vi "Drive Controller.vi"(8 "error in":errorcluster) -> ()   [LabVIEW 2017]
doc: "This VI executes continuously carrying out the current operation and responding to updates or new operation requests. It will often contain the timing or control code that is difficult to place directly in TeleOp. This VI generally opens all sensors and motors and isolates the rest of the robot code from knowing implementation details of how the operations are carried out."
uses:
  Drive Operations.ctl
  Drive Setpoints.ctl
  <vilib>/Rock Robotics/WPI/SafetyOutput/WPI_SafetyOutputConfigMenu.ctl
  <vilib>/Rock Robotics/WPI/RobotDrive/WPI_RobotDriveMecanumDrive_Cartesian.vi
  <vilib>/Rock Robotics/WPI/Framework/Completion Status.ctl
panel:
  in  "Interactive Values":T1
  in  "Buttons":cluster{"Execute Cmd":bool, "Abort Cmd":bool}
  out "Command Timing":cluster{"Start Time (ms)":u32, "Iterations":i32}
  out "Status":T3
  out "Setpoints":T4(graph)
  out "Current\nCmd":string
  # "Tip: The graph shows the motor setpoints. It may also be helpful to observe inputs and sensor values.\nYou may also want to display tuning or debugging controls."
  # "Interactive Command: You may fill in the settings for a command\nand schedule it with the Execute button. You can observe and abort\nany command while fine tuning the code for the controller."
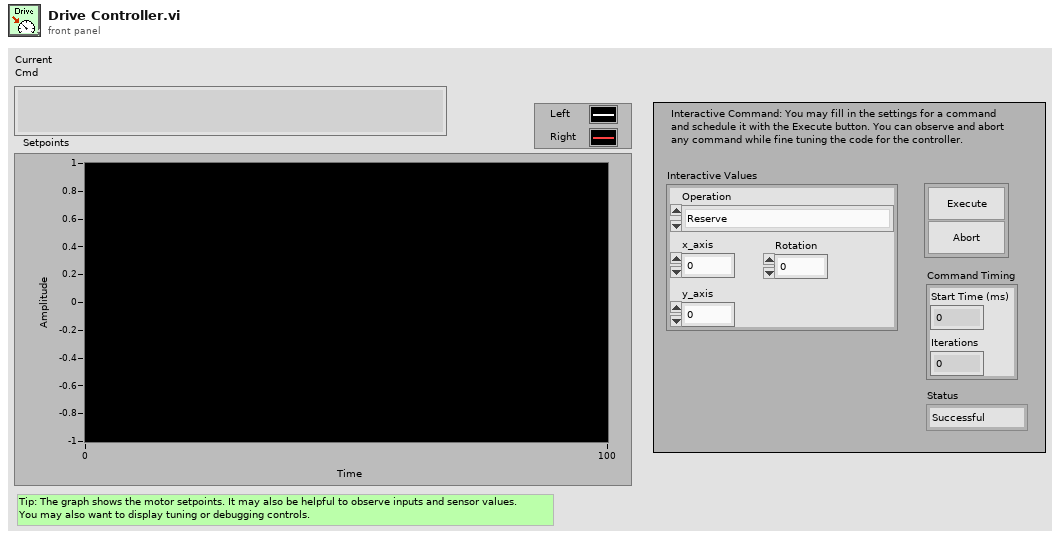
[diagram p1: front panel]
types:
  T1 = typedef "Drive Setpoints.ctl" = cluster{"Operation":T2, "x_axis":dbl, "Rotation":dbl, "y_axis":dbl}
  T2 = typedef "Drive Operations.ctl" = enum16{"Reserve", "Read Current", "Immediate", "Drive for Time", "Drive for Distance"}
  T3 = typedef "Completion Status.ctl" = enum16{"Successful", "Aborted", "Incomplete"}
  T4 = cluster{"Left Setpoint":dbl, "Right Setpoint":dbl}
  T5 = typedef "WPI_SafetyOutputConfigMenu.ctl" = enum16{"Enable", "Disable"}
  T6 = typedef "Command Status Info.ctl" = cluster{"Name":string, "Status":T3, "notifier out":T7}
  T7 = typedef "Completion Notifier.ctl" = refnum<notifier>
  T8 = cluster{"SubSystem Data":T1, cluster{"Start Time (ms)":u32, "Iterations":i32}, cluster{"Command Info":T6, "Description":string, "Default Command":T1, "queue out":refnum<queue>, "Subsystem Name":string}}
  T9 = typedef "WPI_RobotDriveDevRef.ctl" = cluster{"DevStatus":errorcluster, "Motors[]":T10[], "Square Inputs":bool, "Max Output":dbl}
  T10 = typedef "WPI_MotorControlDeviceRef.ctl" = cluster{"DeviceStatus":errorcluster, "Type":T11, "PWM":cluster{"PWM Channel":T12, "DeadBand":T13}, "CAN":cluster{"Device Number":u8, "SetOutput VI Ref":variant, "GetOutput VI Ref":variant, "Enable VI Ref":variant, "Disable VI Ref":variant, "Data":variant}, "Invert":bool, "DIO PWM":cluster{"PWM \"Enable\" Channel":T12, "DIOChannel":T14, "PWM Rate":dbl}}
  T11 = typedef "WPI_MotorControlType.ctl" = enum16{"PWM", "CAN", "DIO PWM"}
  T12 = typedef "FPGA_DIOPWMChannel.ctl" = enum8{"PWM 0", "PWM 1", "PWM 2", "PWM 3", "PWM 4", "PWM 5", "PWM 6", "PWM 7", "PWM 8", "PWM 9", "PWM MXP 0", "PWM MXP 1", "PWM MXP 2", "PWM MXP 3", "PWM MXP 4", "PWM MXP 5", "PWM MXP 6", "PWM MXP 7", "PWM MXP 8", "PWM MXP 9", "Invalid"}
  T13 = typedef "WPI_PWMDeadband.ctl" = cluster{"Name":string, "maxPositivePwm":i32, "minPositivePwm":i32, "centerPwm":i32, "maxNegativePwm":i32, "minNegativePwm":i32, "angularRange":u16}
  T14 = typedef "FPGA_DIOChannel.ctl" = enum8{"DIO 0", "DIO 1", "DIO 2", "DIO 3", "DIO 4", "DIO 5", "DIO 6", "DIO 7", "DIO 8", "DIO 9", "DIO MXP 0", "DIO MXP 1", "DIO MXP 2", "DIO MXP 3", "DIO MXP 4", "DIO MXP 5", "DIO MXP 6", "DIO MXP 7", "DIO MXP 8", "DIO MXP 9", "DIO MXP 10", "DIO MXP 11", "DIO MXP 12", "DIO MXP 13", "DIO MXP 14", "DIO MXP 15", "SPI Port CS1", "SPI Port CS2", "SPI Port CS3", "SPI Port MISO", "SPI Port MOSI", "Invalid"}
  T15 = cluster{"SubSystem Data":T1, cluster{"Start Time (ms)":u32, "Iterations":i32}, "Default Command Arguments":cluster{"Command Info":T6, "Description":string, "Default Command":T1, "queue out":refnum<queue>, "Subsystem Name":string}}
  T16 = cluster{"Don't move motors while reserved":dbl, "Don't move motors while reserved":dbl}
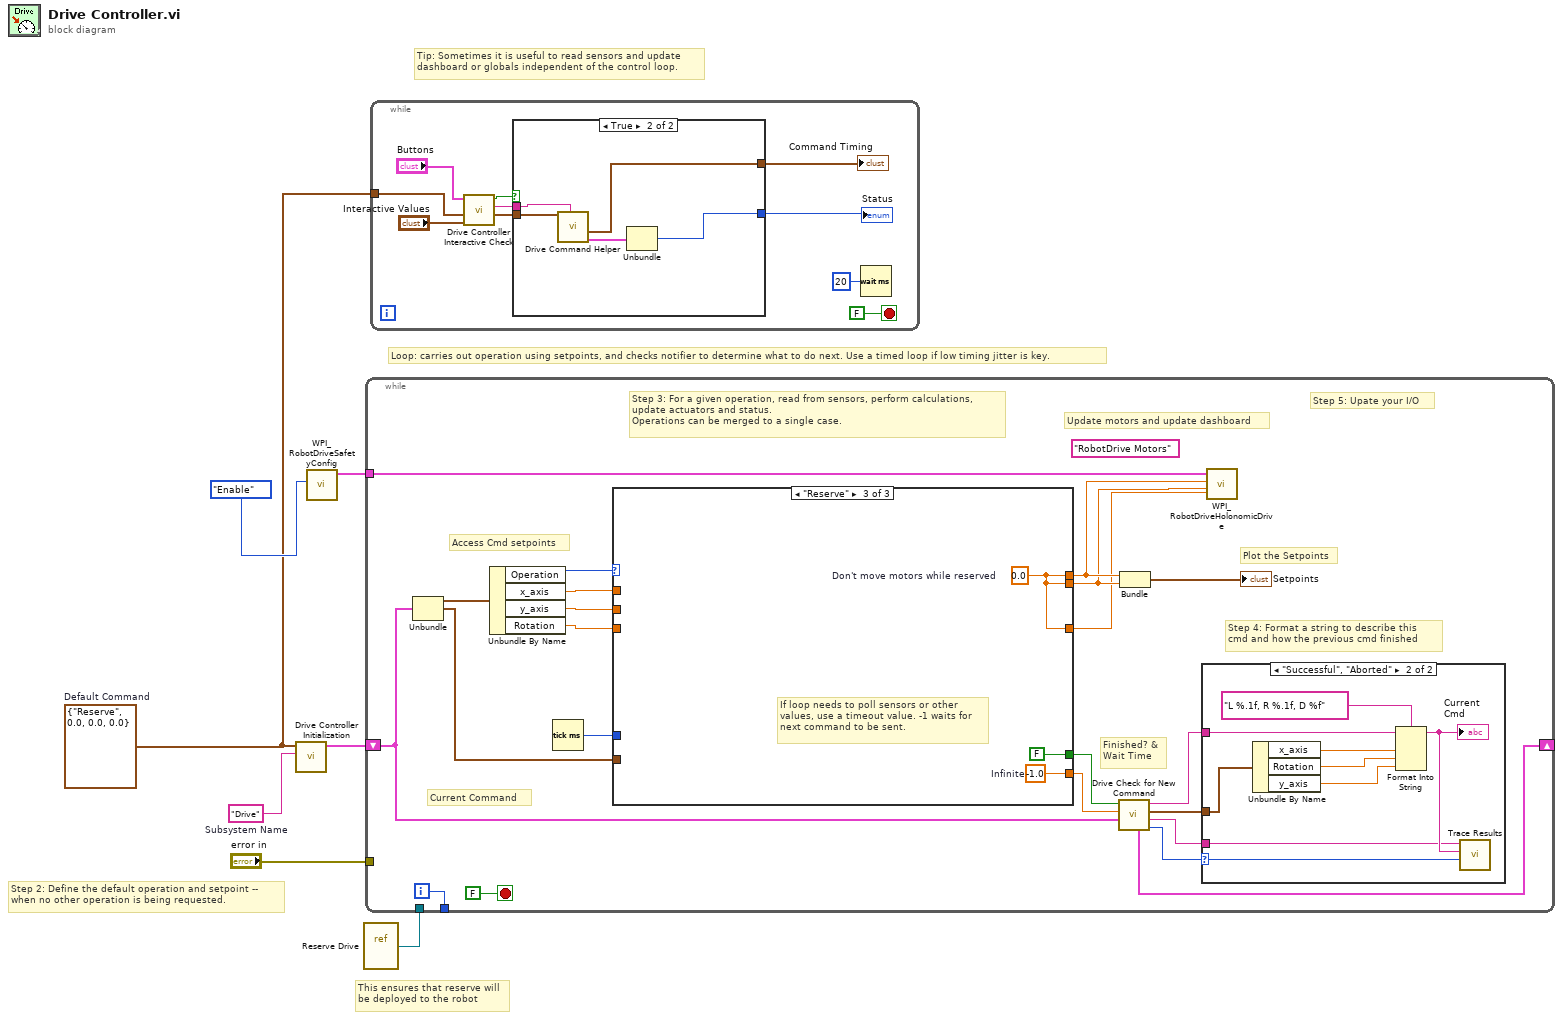
[diagram p0: block diagram]
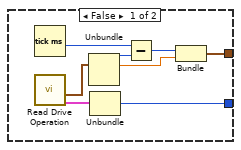
[diagram p2: hidden frame]
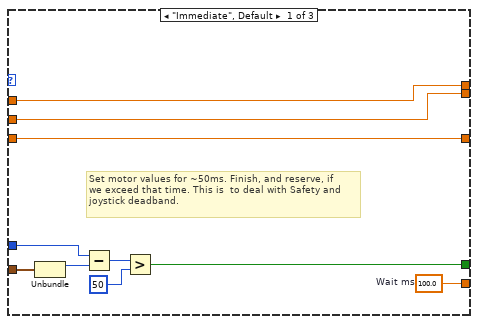
[diagram p4: hidden frame]
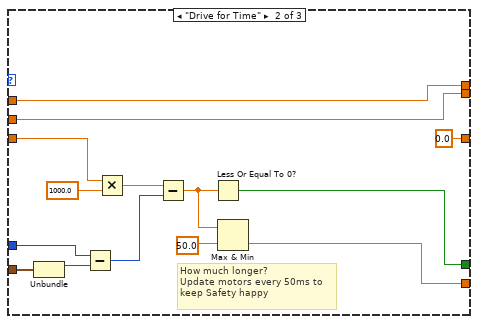
[diagram p5: hidden frame]
diagram:
  w2 = T1 {"Operation"=enum."Reserve", "x_axis"=0.0, "Rotation"=0.0, "y_axis"=0.0}  # Default Command
  w8 = "Drive"  # Subsystem Name
  # "This ensures that reserve will\nbe deployed to the robot"
  # "Tip: Sometimes it is useful to read sensors and update\ndashboard or globals independent of the control loop."
  # "Step 2: Define the default operation and setpoint --\nwhen no other operation is being requested."
  # "Loop: carries out operation using setpoints, and checks notifier to determine what to do next. Use a timed loop if low timing jitter is key."
  n1 = call "Drive Controller Initialization.vi"("Subsystem Name"=w8, "Default Command"=w2) -> ("Current Command"=w4:T8)  [unwired: 9 in]
  n2 = call <vilib>:"WPI_RobotDriveSafetyConfig.vi"("mode"=WPI_SafetyOutputConfigMenu."Enable") -> (3:"RobotDriveDevRef"=w6:T9, 11:"RobotDriveDevRef"=w1:T9)  [unwired: 8 in, 1 out]
  n3 = vi-ref "Reserve Drive.vi"() -> (w3:refnum<vi>)
  n4 = while {
    shift-right: [w20] -> _
    shift-left: w4 -> [w13]
    tunnel: [w29] -> _
    tunnel: w6 -> [w12]
    tunnel: "error in" -> [_]
    tunnel: w3 -> [_]
    i -> [w29]
    stop <- FALSE stop-if-true
    (unwired) "RobotDrive Motors" ("Name")
    # "Step 5: Upate your I/O"
    # "Step 4: Format a string to describe this\ncmd and how the previous cmd finished"
    # "Current Command"
    # "Update motors and update dashboard"
    # "Plot the Setpoints"
    # "Access Cmd setpoints"
    # "Finished? &\nWait Time"
    # "Step 3: For a given operation, read from sensors, perform calculations,\nupdate actuators and status.\nOperations can be merged to a single case."
    n5 = Unbundle(w13) -> ("SubSystem Data"=w27:T1, w14:cluster{"Start Time (ms)":u32, "Iterations":i32})  [unwired: 1 out]
    n6 = Unbundle By Name(w27) -> ("Operation"=w26:T2, "x_axis"=w25:dbl, "y_axis"=w24:dbl, "Rotation"=w23:dbl)
    n7 = Tick Count (ms)() -> (millisecond timer value=w22:u32)
    n8 = case shown="\"Reserve\"" w26 {
      tunnel: [w49 w51 w66] -> w19
      tunnel: [w42 w58 FALSE ("ignore previous (F)")] -> w18
      tunnel: w14 -> [w41 w60 _]
      tunnel: [w48 w57 w64] -> w11
      tunnel: [w47 w56 w64] -> w10
      tunnel: w25 -> [w48 w57 _]
      tunnel: w24 -> [w47 w56 _]
      tunnel: w23 -> [w40 w55 _]
      tunnel: w22 -> [w43 w54 _]
      tunnel: [w40 0.0 ("Rotation") w64] -> w9
      frame "Immediate", Default {
        w49 = 100.0  # Wait ms
        # "Set motor values for ~50ms. Finish, and reserve, if\nwe exceed that time. This is  to deal with Safety and\njoystick deadband."
        n9 = Unbundle(w41) -> ("Start Time (ms)"=w44:u32)  [unwired: 1 out]
        n10 = Subtract(x=w43, y=w44) -> (x-y=w45:u32)
        n11 = Greater?(x=w45, y=u8 50 ("Left Motor")) -> (0:w42:bool)
      }
      frame "Drive for Time" {
        # "How much longer?\nUpdate motors every 50ms to\nkeep Safety happy"
        n12 = Unbundle(w60) -> ("Start Time (ms)"=w59:u32)  [unwired: 1 out]
        n13 = Subtract(x=w54, y=w59) -> (x-y=w63:u32)
        n14 = Multiply(x=w55, y=1000.0) -> (x*y=w62:dbl)
        n15 = Subtract(x=w62, y=w63) -> (x-y=w53:dbl)
        n16 = Less Or Equal To 0?(x=w53) -> (x <= 0?=w58:bool)
        n17 = Max & Min(x=w53, y=50.0) -> (min(x,y)=w51:dbl)  [unwired: 1 out]
      }
      frame "Reserve" {
        w64 = 0.0  # Don't move motors while reserved
        w66 = -1.0  # Infinite
        # "If loop needs to poll sensors or other\nvalues, use a timeout value. -1 waits for\nnext command to be sent."
      }
    }
    n18 = call "Drive Check for New Command.vi"("input cluster"=w13, "Wait time (ms)"=w19, "Finished?"=w18) -> ("Completion"=w21:T3, "Subsystem Name"=w15:string, "Current Command"=w16:T1, "Initial Trace String"=w17:string, "Next Command"=w20:T15)  [unwired: 4 in]
    n19 = Bundle("Don't move motors while reserved"=w11, "Don't move motors while reserved"=w10) -> (→"Setpoints":T16)  [unwired: 1 in]
    n20 = case shown="\"Successful\", \"Aborted\"" w21 {
      selector: w21 -> [_ w39]
      tunnel: w17 -> [_ w34]
      tunnel: w16 -> [_ w35]
      tunnel: w15 -> [_ w31]
      frame "Incomplete", Default {
        # "Continuing current command"
      }
      frame "Successful", "Aborted" {
        # "Report and setup for next command"
        n21 = Unbundle By Name(w35) -> ("x_axis"=w37:dbl, "Rotation"=w38:dbl, "y_axis"=w32:dbl)
        n22 = Format Into String(format string="L %.1f, R %.1f, D %f", initial string=w34, w37, w38, w32) -> (resulting string=w33:string)  [unwired: 1 in, 1 out]
        "Current\nCmd" <- w33
        n23 = call <vilib>:"Trace Results.vi"("Status of previous command"=w39, "Description"=w33, "Subsystem"=w31) -> ()  [unwired: 9 in]
      }
    }
    n24 = call-poly <vilib>:"WPI_RobotDriveHolonomicDrive.vi"("Rotation"=w9, "Y"=w10, "X"=w11, "RobotDriveDevRef"=w12) -> ()  [unwired: 5 in, 3 out]
  }
  n25 = while {
    tunnel: w2 -> [w68]
    stop <- FALSE stop-if-true
    n26 = call "Drive Controller Interactive Check.vi"("Interactive Command In"="Interactive Values", "Default Command"=w68, "Buttons"="Buttons") -> ("Interactive Command Out"=w70:T1, "Trace String"=w71:string, "Schedule"=w72:bool)  [unwired: 6 in]
    n27 = case shown="True" w72 {
      tunnel: [w81 w89] -> w73
      tunnel: [w80 w85] -> w74
      tunnel: w71 -> [_ w87]
      tunnel: w70 -> [_ w86]
      frame False {
        n28 = Tick Count (ms)() -> (millisecond timer value=w84:u32)
        n29 = call "Read Drive Operation.vi"() -> ("Command Info"=w78:T6, "SubSystem Data"=w77:T1)  [unwired: 9 in, 1 out]
        n30 = Unbundle(w77) -> ("Operation"=w82:T2, "x_axis"=w79:dbl)  [unwired: 2 out]
        n31 = Unbundle(w78) -> ("Status"=w81:T3)  [unwired: 2 out]
        n32 = Subtract(x=w84, y=w82) -> (x-y=w83:u32)
        n33 = Bundle(w83, "x_axis"=w79) -> (w80:cluster{u32, "x_axis":dbl})  [unwired: 1 in]
      }
      frame True {
        n34 = call "Drive Command Helper.vi"("Description"=w87, "SubSystem Data"=w86) -> ("Command Info Out"=w88:T6, "Command Timing"=w85:cluster{"Start Time (ms)":u32, "Iterations":i32})  [unwired: 7 in, 1 out]
        n35 = Unbundle(w88) -> ("Status"=w89:T3)  [unwired: 2 out]
      }
    }
    "Status" <- w73
    "Command Timing" <- w74
    n36 = Wait (ms)(milliseconds to wait=u32 20) -> ()  [unwired: 1 out]
  }
